vi "禹山溶解氧校准.vi"() -> ()   [LabVIEW 2016, in "斯坦道多参数.lvlib"]
uses:
  <vilib>/Utility/miscctls.llb/LVPointTypeDef.ctl
  <vilib>/Analysis/NI_AALBase.lvlib
  <vilib>/Analysis/NI_AALPro.lvlib
  <vilib>/Utility/config.llb/NI_LVConfig.lvlib
panel:
  in  "盐度自动获取":bool
  in  "大气压补偿":dbl
  in  "盐度补偿":dbl
  out "DO %":dbl caption="饱和度值"
  out "第二点校准值":dbl
  out "第一点校准值":dbl
  out "最小值":sgl format="%.2g"
  out "最大值":sgl format="%.2g"
  in  "校准停止":bool
  in  "校准模式":enum16{"两点校准", "单点校准"}(ring)
  in  "标液2":dbl
  in  "标液1":dbl
  out "波形图表":sgl(graph) caption="历史曲线"
  out "温度测量值":dbl caption="温度"
  out "变异系数":dbl format="%.6g"
  out "standard deviation":dbl caption="标准差" format="%0.2f"
  out "mean":dbl caption="均值" format="%0.2f"
  out "提示":string
  in  "校准启动":bool
  out "DO mg/L":dbl caption="测试值"
  out "电极斜率":dbl
  out "电极零点":dbl
  # "溶解氧电极设定"
  # "℃"
  # "%"
  # "mg/L"
  # "kPa"
  # "请选择校准模式:"
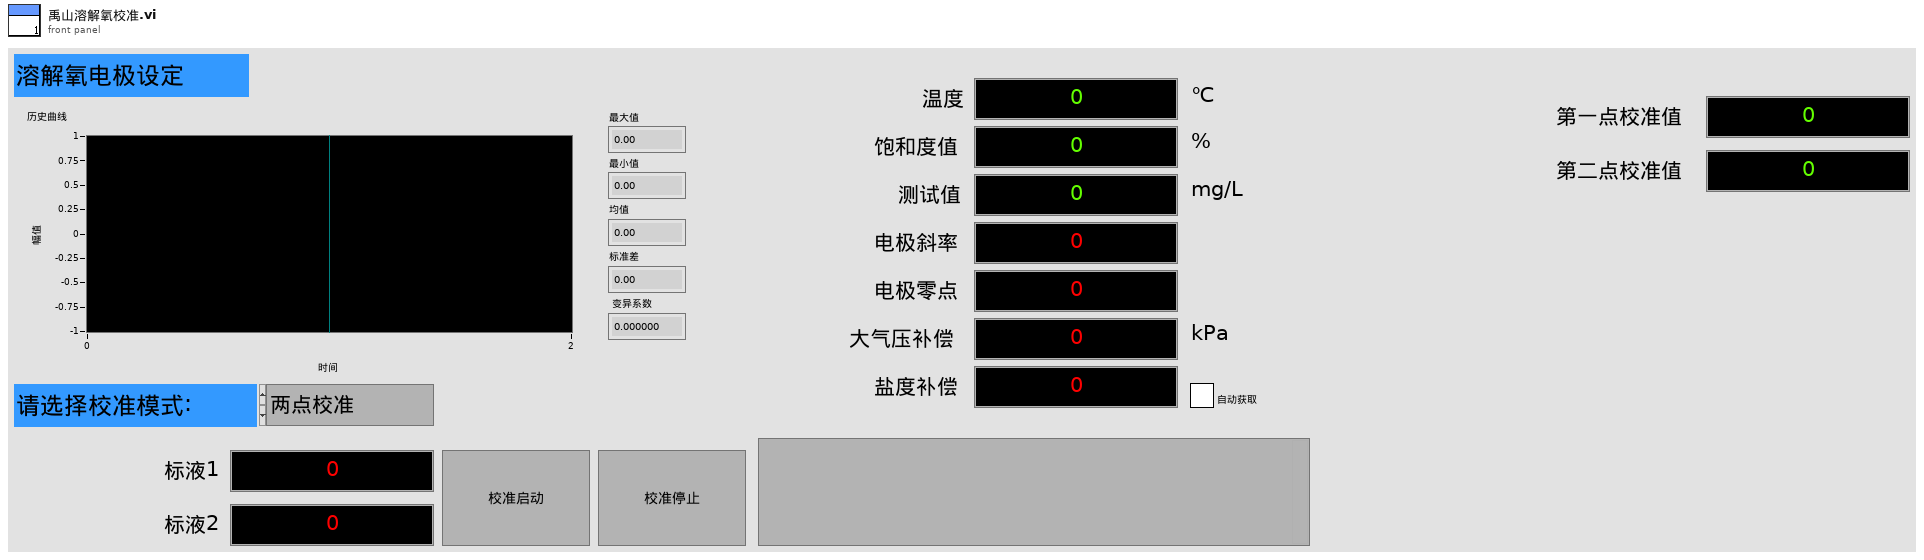
[diagram p1: front panel]
types:
  T1 = typedef "斯坦道多参数.lvlib/校准步骤.ctl" = enum16{"待机", "放置第一点标液", "第一点校准启动", "第一点校准写入", "第一点校准失败", "放置第二点标液", "第二点校准启动", "第二点校准写入", "第二点校准失败", "放置第三点标液", "第三点校准启动", "第三点校准写入", "第三点校准失败", "校准结果写入", "校准结束"}
  T2 = typedef "LVPointTypeDef.ctl" = cluster{"Horizontal":i16, "Vertical":i16}
  T3 = typedef "NI_LVConfig.lvlib/Config Data RefNum.ctl" = refnum<k1>
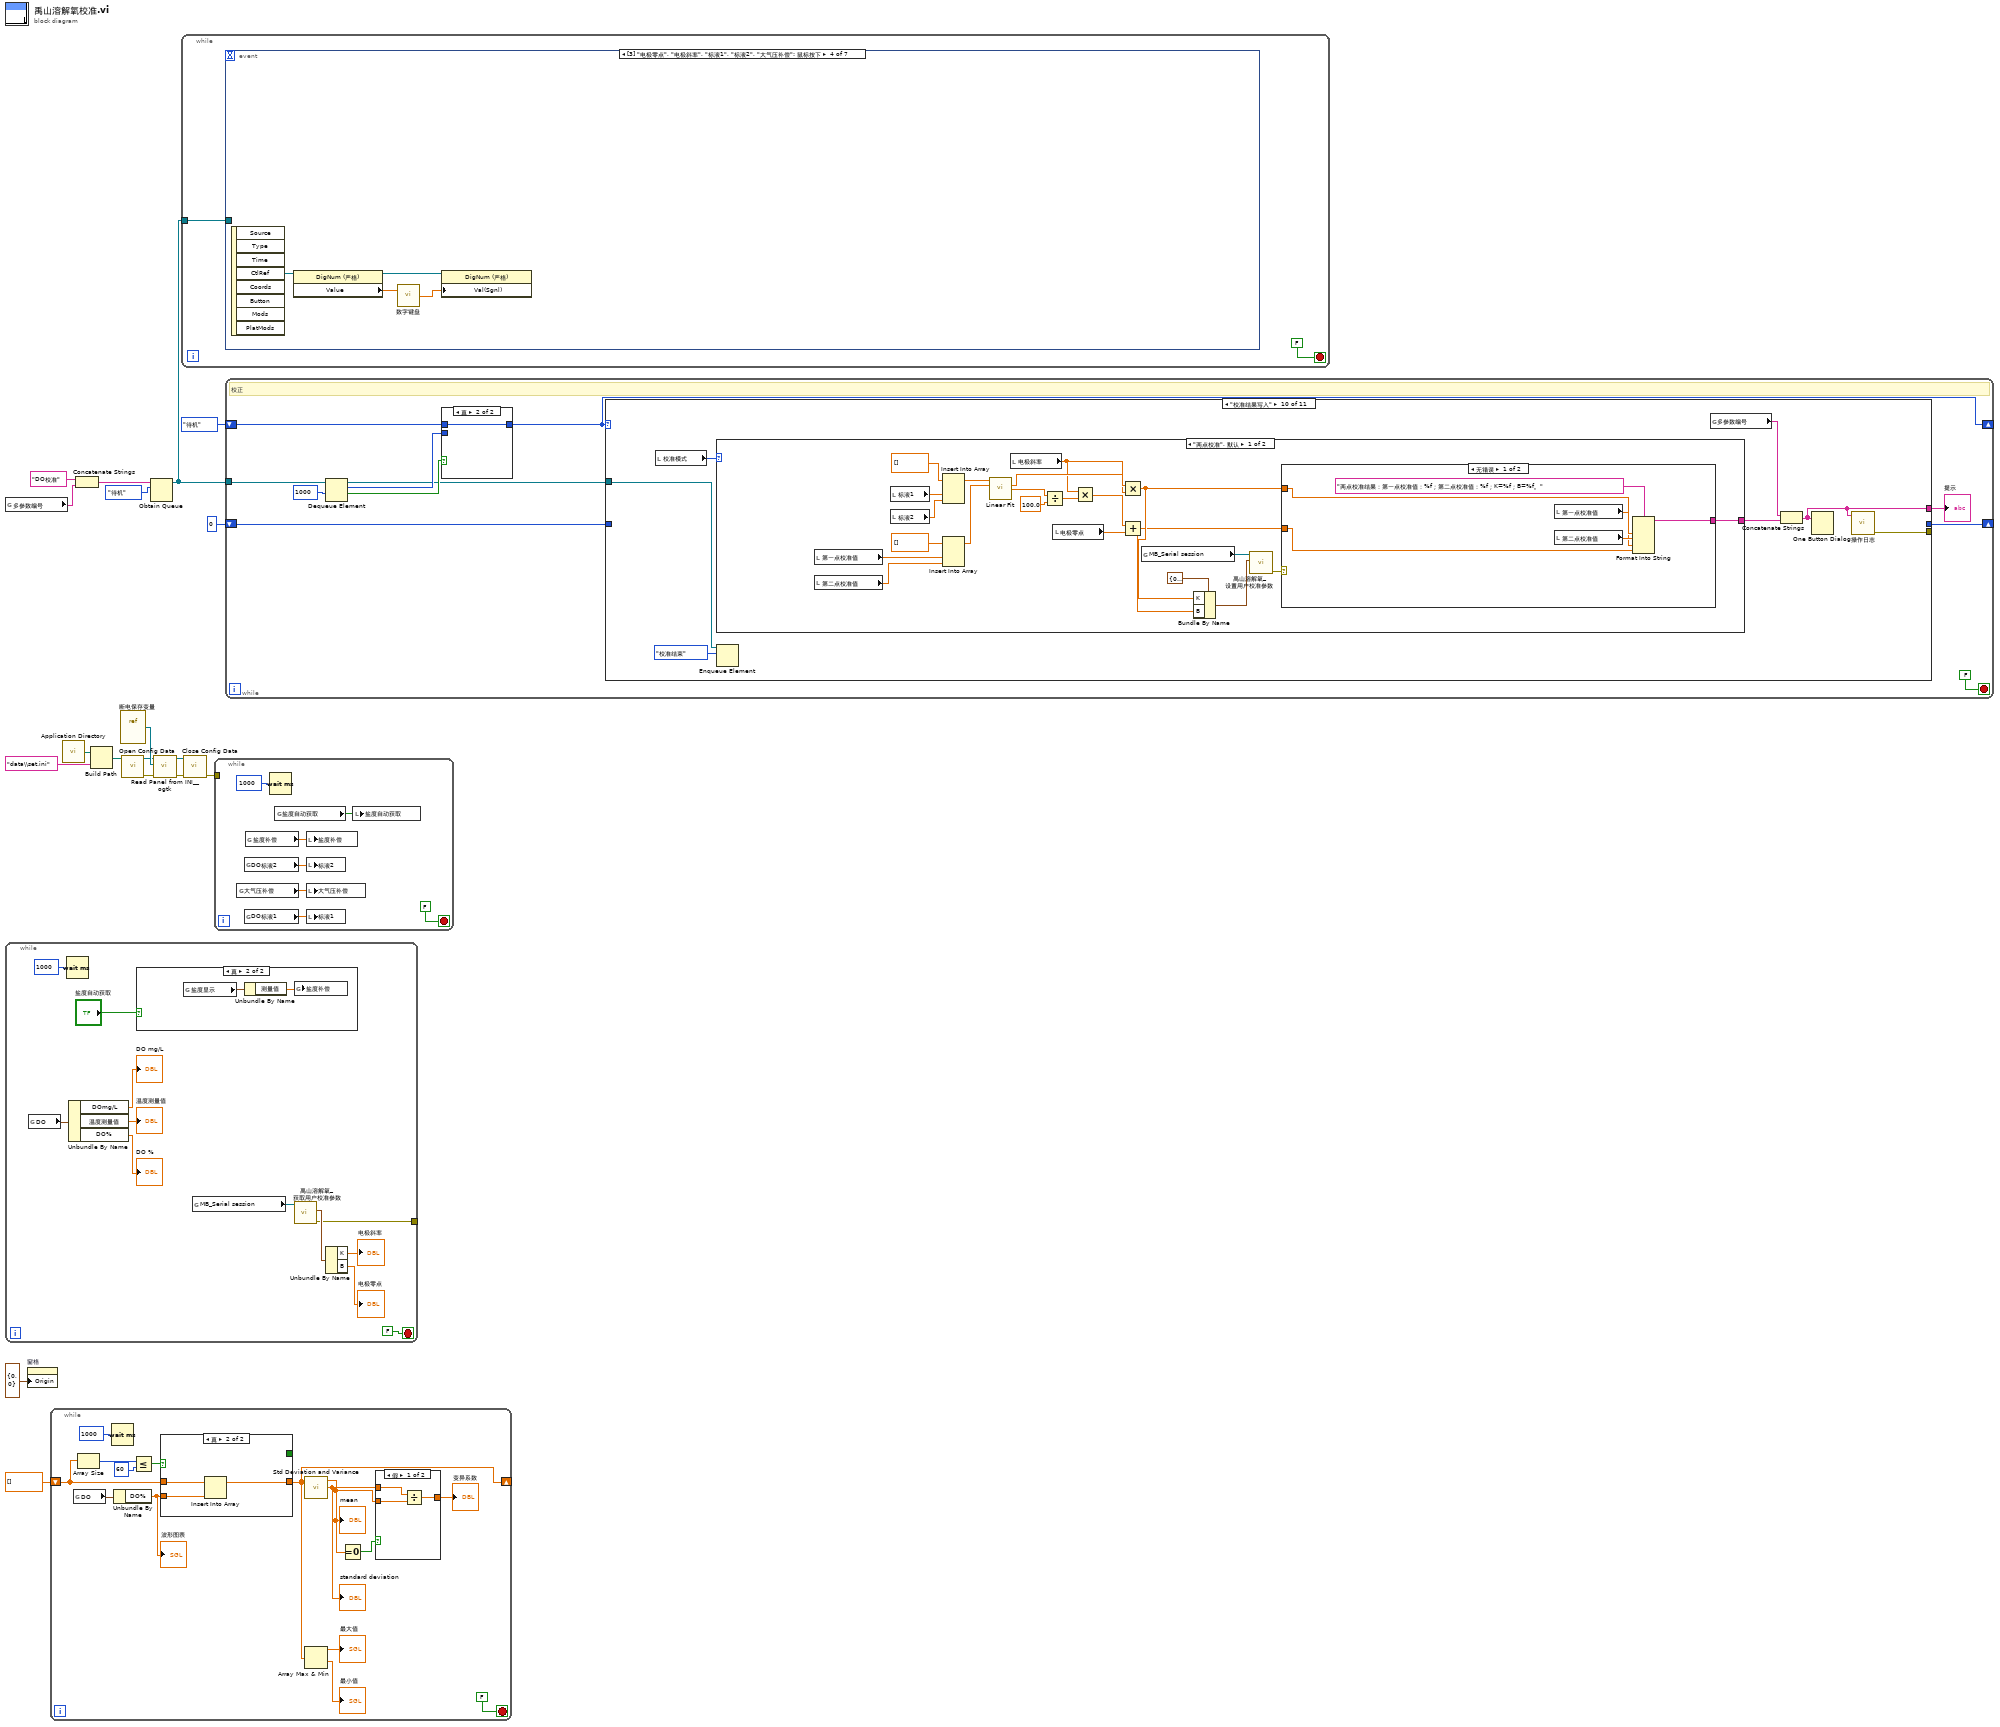
[diagram p0: block diagram]
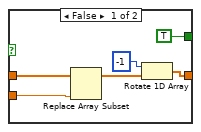
[diagram p3: hidden frame]
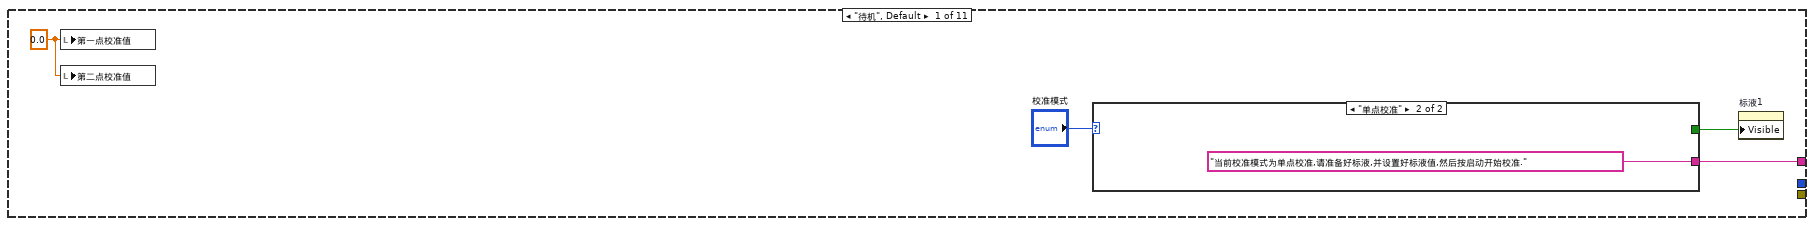
[diagram p5: hidden frame]
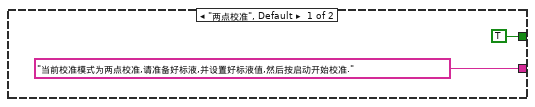
[diagram p6: hidden frame]
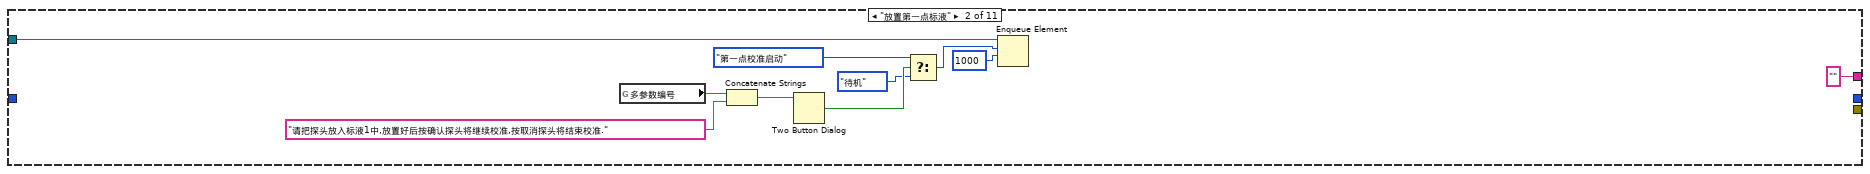
[diagram p7: hidden frame]
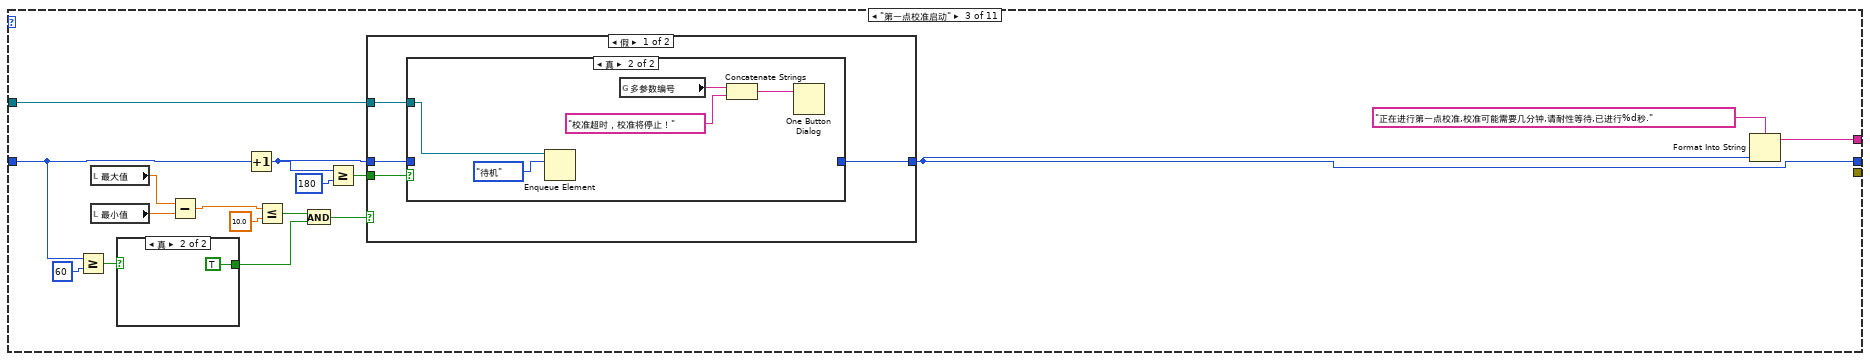
[diagram p8: hidden frame]
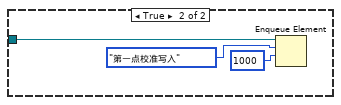
[diagram p10: hidden frame]
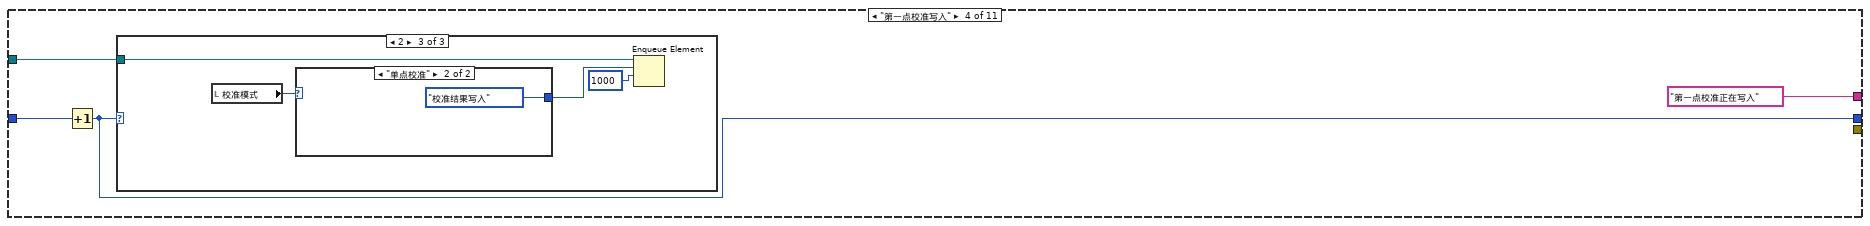
[diagram p12: hidden frame]
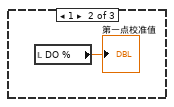
[diagram p14: hidden frame]
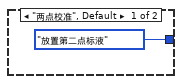
[diagram p15: hidden frame]
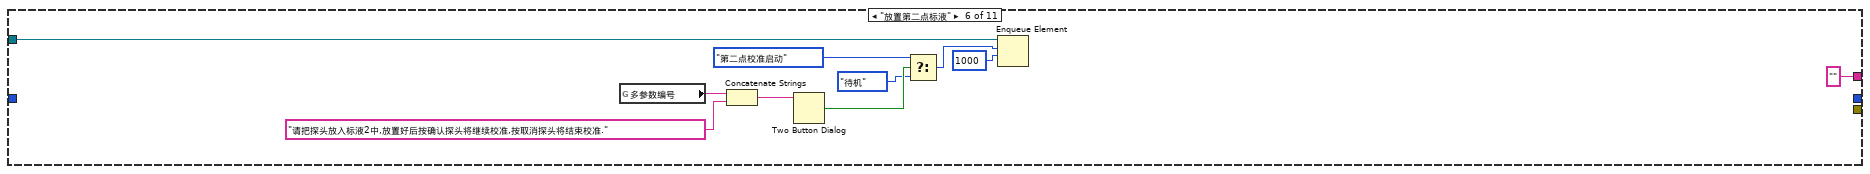
[diagram p17: hidden frame]
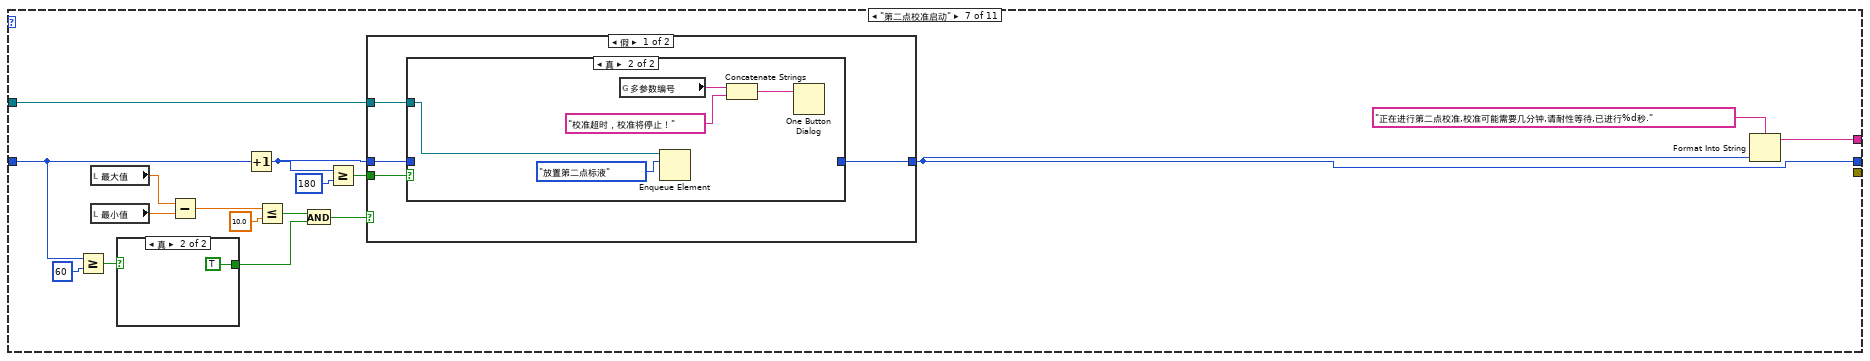
[diagram p18: hidden frame]
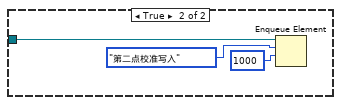
[diagram p20: hidden frame]
diagram:
  n1 = global read "多参数全局变量.vi" "多参数编号"() -> (w1:string)
  n2 = while {
    tunnel: [w25] -> _
    stop <- FALSE stop-if-true
    n3 = global read "禹山过程全局变量.vi" "DO"() -> (w22:cluster{"温度测量值":sgl, "DO%":sgl, "DOmg/L":sgl})
    n4 = Wait (ms)(milliseconds to wait=u32 1000 ("等待时间（毫秒）")) -> ()  [unwired: 1 out]
    n5 = Unbundle By Name(w22) -> ("DOmg/L"=→"DO mg/L":sgl, "温度测量值"=→"温度测量值":sgl, "DO%"=→"DO %":sgl)
    n6 = case shown="真" "盐度自动获取" {
      frame False {
      }
      frame True {
        n7 = global read "多参数全局变量.vi" "盐度显示"() -> (w32:cluster{"温度测量值":sgl, "测量值":sgl, "温度偏移修正值":sgl})
        n8 = Unbundle By Name(w32) -> ("测量值"=w31:sgl)
        n9 = global write "断电保存变量.vi" "盐度补偿"(w31) -> ()
      }
    }
    n10 = global read "多参数全局变量.vi" "MB_Serial session"() -> (w21:refnum<class "MB_Master_Serial.lvclass">)
    n11 = call "禹山溶解氧_获取用户校准参数.vi"("MB_Serial session in"=w21) -> ("error out"=w25:errorcluster, "输出值"=w28:cluster{"K":sgl, "B":sgl})  [unwired: 8 in, 1 out]
    n12 = Unbundle By Name(w28) -> ("K"=→"电极斜率":sgl, "B"=→"电极零点":sgl)
  }
  n13 = property on="窗格" class="Pane"("Origin"=T2 {"Horizontal"=0, "Vertical"=0} ("原点")) -> ()  [unwired: 2 in, 2 out]
  n14 = while {
    shift-right: [w35] -> _
    shift-left: sgl[] [] -> [w43]
    stop <- FALSE stop-if-true
    n15 = global read "禹山过程全局变量.vi" "DO"() -> (w37:cluster{"温度测量值":sgl, "DO%":sgl, "DOmg/L":sgl})
    n16 = Array Size(array=w43) -> (size(s)=w45:i32)
    n17 = Wait (ms)(milliseconds to wait=u32 1000 ("等待时间（毫秒）")) -> ()  [unwired: 1 out]
    n18 = Unbundle By Name(w37) -> ("DO%"=w36:sgl)
    "波形图表" <- w36
    n19 = Less Or Equal?(x=w45, y=60) -> (x <= y?=w44:bool)
    n20 = case shown="真" w44 {
      tunnel: w43 -> [w56 w59]
      tunnel: w36 -> [w54 w58]
      tunnel: [w52 w57] -> w35
      tunnel: [TRUE _] -> _
      frame False {
        n21 = Replace Array Subset(array=w56, new element=w54) -> (w55:sgl[])  [unwired: 1 in]
        n22 = Rotate 1D Array(1:w55, 2:-1 ("n")) -> (0:w52:sgl[])
      }
      frame True {
        n23 = Insert Into Array(array=w59, new element=w58) -> (w57:sgl[])  [unwired: 1 in]
      }
    }
    n24 = call <vilib>:"Std Deviation and Variance.vi"("X"=w35) -> ("mean"=w38:dbl, "standard deviation"=w39:dbl)  [unwired: 1 in, 1 out]
    "standard deviation" <- w39
    "mean" <- w38
    n25 = Array Max & Min(array=w35) -> (max value=→"最大值":sgl, min value=→"最小值":sgl)  [unwired: 2 out]
    n26 = Equal To 0?(x=w38) -> (x = 0?=w42:bool)
    n27 = case shown="假" w42 {
      tunnel: w39 -> [w50 _]
      tunnel: [w49 _] -> w41
      tunnel: w38 -> [w48 _]
      frame False {
        n28 = Divide(x=w50, y=w48) -> (x/y=w49:dbl)
      }
      frame True {
      }
    }
    "变异系数" <- w41
  }
  n29 = call <vilib>:"Application Directory.vi"() -> ("Application Directory"=w9:path)
  n30 = Concatenate Strings("DO校准" ("名称（未命名）"), w1) -> (w2:string)
  n31 = Build Path(base path=w9, name or relative path="data\\set.ini" ("名称或相对路径")) -> (appended path=w10:path)
  n32 = vi-ref "断电保存变量.vi"() -> (w12:refnum<vi>)
  n33 = call <vilib>:"Open Config Data.vi"("configuration file path"=w10) -> ("error out"=w6:errorcluster, "refnum"=w5:T3)  [unwired: 8 in, 1 out]
  n34 = Obtain Queue(name (unnamed)=w2, element data type=校准步骤."待机" ("枚举")) -> (queue out=w13:refnum<queue>)  [unwired: 3 in, 2 out]
  n35 = call <userlib>:"Read Panel from INI__ogtk.vi"("error in (no error)"=w6, "VI ref"=w12, "refnum"=w5) -> ("error out"=w8:errorcluster, "refnum out"=w7:T3)  [unwired: 7 in]
  n36 = while {
    tunnel: w13 -> [w60]
    stop <- FALSE stop-if-true
    n37 = event shown="[3] \"电极零点\", \"电极斜率\", \"标液1\", \"标液2\", \"大气压补偿\": 鼠标按下" {
      selector: _ -> [_ _ _ _ _ _ _]
      dyn-events: _ -> [_ _ _ _ _ _ _]
      timeout: _ -> [_ _ _ _ _ _ _]
      tunnel: w60 -> [_ w64 w70 _ _ _ _]
      event Timeout {
        n38 = event-data() -> ()  [unwired: 1 in, 3 out]
      }
      event "校准启动": Value Change {
        n39 = event-data() -> ()  [unwired: 1 in, 6 out]
        n40 = local read "校准模式"() -> (w63:enum16{"两点校准", "单点校准"})
        n41 = case shown="\"两点校准\", 默认" w63 {
          tunnel: [校准步骤."放置第一点标液" ("元素") 校准步骤."放置第二点标液" ("元素")] -> w62
          frame "两点校准", Default {
          }
          frame "单点校准" {
          }
        }
        n42 = Enqueue Element(queue=w64, element=w62) -> ()  [unwired: 2 in, 3 out]
      }
      event "校准停止": Value Change {
        n43 = event-data() -> ()  [unwired: 1 in, 6 out]
        n44 = Flush Queue(queue=w70) -> (queue out=w67:refnum<queue>)  [unwired: 1 in, 2 out]
        n45 = Enqueue Element(queue=w67, element=校准步骤."待机" ("元素"), timeout in ms (-1)=1000 ("超时毫秒(-1)")) -> ()  [unwired: 1 in, 3 out]
      }
      event "电极零点", "电极斜率", "标液1", "标液2", "大气压补偿": Mouse Down {
        n46 = event-data() -> ("CtlRef"=w71:refnum<vi>)  [unwired: 1 in, 7 out]
        n47 = property class="DigNum (严格)"(reference=w71) -> (reference out=w72:refnum<vi>, "Value"=w73:dbl)  [unwired: 1 in, 1 out]
        n48 = call "数字键盘.vi"("OldNumber"=w73) -> ("NewNumber"=w74:dbl)  [unwired: 1 in]
        n49 = property class="DigNum (严格)"(reference=w72, "Val(Sgnl)"=w74) -> ()  [unwired: 1 in, 2 out]
      }
      event "盐度补偿": Mouse Down {
        n50 = event-data() -> ("CtlRef"=w76:refnum<vi>)  [unwired: 1 in, 7 out]
        n51 = local read "盐度自动获取"() -> (w75:bool)
        n52 = case shown="假" w75 {
          tunnel: w76 -> [w77 _]
          frame False {
            n53 = property class="DigNum (严格)"(reference=w77) -> (reference out=w78:refnum<vi>, "Value"=w79:dbl)  [unwired: 1 in, 1 out]
            n54 = call "数字键盘.vi"("OldNumber"=w79) -> ("NewNumber"=w80:dbl)  [unwired: 1 in]
            n55 = property class="DigNum (严格)"(reference=w78, "Val(Sgnl)"=w80) -> ()  [unwired: 1 in, 2 out]
          }
          frame True {
          }
        }
      }
      event "电极零点", "电极斜率": Value Change {
        n56 = event-data() -> ()  [unwired: 1 in, 6 out]
        n57 = local read "电极斜率"() -> (w83:dbl)
        n58 = local read "电极零点"() -> (w82:dbl)
        n59 = global read "多参数全局变量.vi" "MB_Serial session"() -> (w81:refnum<class "MB_Master_Serial.lvclass">)
        n60 = Bundle By Name(cluster=cluster{"K":sgl, "B":sgl} {"K"=0.0, "B"=0.0} ("用户校准参数"), "K"=w83, "B"=w82) -> (w84:cluster{"K":sgl, "B":sgl})
        n61 = call "禹山溶解氧_设置用户校准参数.vi"("用户校准参数"=w84, "MB_Serial session in"=w81) -> ()  [unwired: 8 in, 2 out]
      }
      event "标液1", "标液2", "盐度补偿", "大气压补偿", "盐度自动获取": Value Change {
        n62 = event-data() -> ()  [unwired: 1 in, 6 out]
        n63 = flat-sequence {
          frame #0 {
            n64 = local read "盐度自动获取"() -> (w86:bool)
            n65 = global write "断电保存变量.vi" "DO标液2"("标液2") -> ()
            n66 = global write "断电保存变量.vi" "盐度补偿"("盐度补偿") -> ()
            n67 = global write "断电保存变量.vi" "DO标液1"("标液1") -> ()
            n68 = global write "断电保存变量.vi" "大气压补偿"("大气压补偿") -> ()
            n69 = global write "断电保存变量.vi" "盐度自动获取"(w86) -> ()
          }
          frame #1 {
            n70 = call <vilib>:"Application Directory.vi"() -> ("Application Directory"=w100:path)
            n71 = Build Path(base path=w100, name or relative path="data\\set.ini" ("名称或相对路径")) -> (appended path=w99:path)
            n72 = call <vilib>:"Open Config Data.vi"("configuration file path"=w99) -> ("error out"=w103:errorcluster, "refnum"=w104:T3)  [unwired: 8 in, 1 out]
            n73 = vi-ref "断电保存变量.vi"() -> (w97:refnum<vi>)
            n74 = call <userlib>:"Write Panel to INI__ogtk.vi"("error in (no error)"=w103, "VI ref"=w97, "refnum"=w104) -> ("error out"=w101:errorcluster, "refnum out"=w102:T3)  [unwired: 7 in]
            n75 = call <vilib>:"Close Config Data.vi"("error in (no error)"=w101, "refnum"=w102) -> ("error out"=w93:errorcluster, "file path"=w94:path)  [unwired: 8 in]
            n76 = Open/Create/Replace File(file path (use dialog)=w94, error in=w93) -> (refnum out=w95:refnum<file>, error out=w96:errorcluster)  [unwired: 4 in, 1 out]
            n77 = Flush File(refnum=w95, error in=w96) -> (refnum out=w91:refnum<file>, error out=w92:errorcluster)
            n78 = Close File(refnum=w91, error in=w92) -> ()  [unwired: 2 out]
          }
        }
      }
    }
  }
  n79 = call <vilib>:"Close Config Data.vi"("error in (no error)"=w8, "refnum"=w7) -> ("error out"=w4:errorcluster)  [unwired: 8 in, 1 out]
  n80 = while {
    tunnel: w4 -> [_]
    stop <- FALSE stop-if-true
    n81 = global read "断电保存变量.vi" "大气压补偿"() -> (w107:dbl)
    n82 = global read "断电保存变量.vi" "DO标液2"() -> (w108:dbl)
    n83 = global read "断电保存变量.vi" "DO标液1"() -> (w109:dbl)
    n84 = global read "断电保存变量.vi" "盐度补偿"() -> (w105:dbl)
    n85 = Wait (ms)(milliseconds to wait=u32 1000 ("等待时间（毫秒）")) -> ()  [unwired: 1 out]
    n86 = global read "断电保存变量.vi" "盐度自动获取"() -> (w106:bool)
    n87 = local write "盐度补偿"(w105) -> ()
    n88 = local write "标液2"(w108) -> ()
    n89 = local write "大气压补偿"(w107) -> ()
    n90 = local write "标液1"(w109) -> ()
    n91 = local write "盐度自动获取"(w106) -> ()
  }
  n92 = while "While循环" {
    shift-right: [w113] -> _
    shift-left: 校准步骤."待机" ("枚举") -> [w114]
    shift-right: [w120] -> _
    shift-left: 0 -> [w121]
    tunnel: w13 -> [w118]
    stop <- FALSE stop-if-true
    # "校正"
    n93 = Dequeue Element(queue=w118, timeout in ms (-1)=1000 ("超时毫秒(-1)")) -> (queue out=w112:refnum<queue>, element=w115:T1, timed out?=w116:bool)  [unwired: 1 in, 1 out]
    n94 = case shown="真" w116 {
      tunnel: w115 -> [w123 _]
      tunnel: [w123 w124] -> w113
      tunnel: w114 -> [_ w124]
      frame False {
      }
      frame True {
      }
    }
    n95 = case shown="\"校准结果写入\"" w113 {
      tunnel: [w128 "" ("提示") w157 "第一点校准正在写入" ("提示") _ "" ("提示") w209 "第二点校准正在写入" ("提示") _ w234 w286] -> w119
      tunnel: w121 -> [_ _ w151 w175 _ _ w203 w227 _ _ _]
      tunnel: [_ _ w142 w174 _ _ w194 w226 _ _ _] -> w120
      tunnel: w112 -> [_ w140 w145 w173 _ w192 w197 w225 _ w238 _]
      tunnel: [_ _ _ _ _ _ _ _ _ w233 _] -> _
      frame "待机", Default {
        w125 = 0.0 ("第一点校准值")
        n96 = local write "第一点校准值"(w125) -> ()
        n97 = local write "第二点校准值"(w125) -> ()
        n98 = case shown="\"单点校准\"" "校准模式" {
          tunnel: ["当前校准模式为两点校准,请准备好标液,并设置好标液值,然后按启动开始校准." ("提示") "当前校准模式为单点校准,请准备好标液,并设置好标液值,然后按启动开始校准." ("提示")] -> w128
          tunnel: [TRUE ("可见") _] -> w126
          frame "两点校准", Default {
          }
          frame "单点校准" {
          }
        }
        n99 = property on="标液1" class="DigNum (严格)"("Visible"=w126) -> ()  [unwired: 2 in, 2 out]
      }
      frame "放置第一点标液" {
        n100 = global read "多参数全局变量.vi" "多参数编号"() -> (w132:string)
        n101 = Concatenate Strings(w132, "请把探头放入标液1中,放置好后按确认探头将继续校准,按取消探头将结束校准." ("消息")) -> (w133:string)
        n102 = Two Button Dialog(message=w133) -> (T button?=w138:bool)  [unwired: 2 in]
        n103 = Select(t=校准步骤."第一点校准启动" ("元素"), s=w138, f=校准步骤."待机" ("元素")) -> (s? t:f=w135:T1)
        n104 = Enqueue Element(queue=w140, element=w135, timeout in ms (-1)=1000 ("超时毫秒(-1)")) -> ()  [unwired: 1 in, 3 out]
      }
      frame "第一点校准启动" {
        n105 = Greater Or Equal?(x=w151, y=60) -> (x >= y?=w152:bool)
        n106 = local read "最大值"() -> (w148:sgl)
        n107 = local read "最小值"() -> (w149:sgl)
        n108 = case shown="真" w152 {
          tunnel: [_ TRUE] -> w150
          frame False {
          }
          frame True {
          }
        }
        n109 = Subtract(x=w148, y=w149) -> (x-y=w147:sgl)
        n110 = Increment(x=w151) -> (x+1=w143:i32)
        n111 = Less Or Equal?(x=w147, y=10.0) -> (x <= y?=w155:bool)
        n112 = And(x=w155, y=w150) -> (x .and. y?=w146:bool)
        n113 = Greater Or Equal?(x=w143, y=180) -> (x >= y?=w144:bool)
        n114 = case shown="假" w146 {
          tunnel: w145 -> [w161 w171]
          tunnel: w144 -> [w162 _]
          tunnel: w143 -> [w160 _]
          tunnel: [w159 _] -> w142
          frame False {
            n115 = case shown="真" w162 {
              tunnel: w161 -> [_ w168]
              tunnel: w160 -> [w163 _]
              tunnel: [w163 _] -> w159
              frame False {
              }
              frame True {
                n116 = Enqueue Element(queue=w168, element=校准步骤."待机" ("元素")) -> ()  [unwired: 2 in, 3 out]
                n117 = global read "多参数全局变量.vi" "多参数编号"() -> (w164:string)
                n118 = Concatenate Strings(w164, "校准超时，校准将停止！" ("消息")) -> (w165:string)
                n119 = One Button Dialog(message=w165) -> ()  [unwired: 1 in, 1 out]
              }
            }
          }
          frame True {
            n120 = Enqueue Element(queue=w171, element=校准步骤."第一点校准写入" ("元素"), timeout in ms (-1)=1000 ("超时毫秒(-1)")) -> ()  [unwired: 1 in, 3 out]
          }
        }
        n121 = Format Into String(format string="正在进行第一点校准,校准可能需要几分钟,请耐性等待,已进行%d秒." ("格式字符串"), w142) -> (resulting string=w157:string)  [unwired: 2 in, 1 out]
      }
      frame "第一点校准写入" {
        n122 = Increment(x=w175) -> (x+1=w174:i32)
        n123 = case shown="2" w174 {
          tunnel: w173 -> [_ _ w181]
          frame 0, Default {
          }
          frame 1 {
            n124 = local read "DO %"() -> (→"第一点校准值":dbl)
          }
          frame 2 {
            n125 = local read "校准模式"() -> (w180:enum16{"两点校准", "单点校准"})
            n126 = case shown="\"单点校准\"" w180 {
              tunnel: [校准步骤."放置第二点标液" ("元素") 校准步骤."校准结果写入" ("元素")] -> w179
              frame "两点校准", Default {
              }
              frame "单点校准" {
              }
            }
            n127 = Enqueue Element(queue=w181, element=w179, timeout in ms (-1)=1000 ("超时毫秒(-1)")) -> ()  [unwired: 1 in, 3 out]
          }
        }
      }
      frame "第一点校准失败" {
      }
      frame "放置第二点标液" {
        n128 = global read "多参数全局变量.vi" "多参数编号"() -> (w184:string)
        n129 = Concatenate Strings(w184, "请把探头放入标液2中,放置好后按确认探头将继续校准,按取消探头将结束校准." ("消息")) -> (w185:string)
        n130 = Two Button Dialog(message=w185) -> (T button?=w190:bool)  [unwired: 2 in]
        n131 = Select(t=校准步骤."第二点校准启动" ("元素"), s=w190, f=校准步骤."待机" ("元素")) -> (s? t:f=w187:T1)
        n132 = Enqueue Element(queue=w192, element=w187, timeout in ms (-1)=1000 ("超时毫秒(-1)")) -> ()  [unwired: 1 in, 3 out]
      }
      frame "第二点校准启动" {
        n133 = Greater Or Equal?(x=w203, y=60) -> (x >= y?=w204:bool)
        n134 = local read "最大值"() -> (w200:sgl)
        n135 = local read "最小值"() -> (w201:sgl)
        n136 = case shown="真" w204 {
          tunnel: [_ TRUE] -> w202
          frame False {
          }
          frame True {
          }
        }
        n137 = Subtract(x=w200, y=w201) -> (x-y=w199:sgl)
        n138 = Increment(x=w203) -> (x+1=w195:i32)
        n139 = Less Or Equal?(x=w199, y=10.0) -> (x <= y?=w207:bool)
        n140 = And(x=w207, y=w202) -> (x .and. y?=w198:bool)
        n141 = Greater Or Equal?(x=w195, y=180) -> (x >= y?=w196:bool)
        n142 = case shown="假" w198 {
          tunnel: w197 -> [w213 w223]
          tunnel: w196 -> [w214 _]
          tunnel: w195 -> [w212 _]
          tunnel: [w211 _] -> w194
          frame False {
            n143 = case shown="真" w214 {
              tunnel: w213 -> [_ w220]
              tunnel: w212 -> [w215 _]
              tunnel: [w215 _] -> w211
              frame False {
              }
              frame True {
                n144 = global read "多参数全局变量.vi" "多参数编号"() -> (w216:string)
                n145 = Enqueue Element(queue=w220, element=校准步骤."放置第二点标液" ("元素")) -> ()  [unwired: 2 in, 3 out]
                n146 = Concatenate Strings(w216, "校准超时，校准将停止！" ("消息")) -> (w217:string)
                n147 = One Button Dialog(message=w217) -> ()  [unwired: 1 in, 1 out]
              }
            }
          }
          frame True {
            n148 = Enqueue Element(queue=w223, element=校准步骤."第二点校准写入" ("元素"), timeout in ms (-1)=1000 ("超时毫秒(-1)")) -> ()  [unwired: 1 in, 3 out]
          }
        }
        n149 = Format Into String(format string="正在进行第二点校准,校准可能需要几分钟,请耐性等待,已进行%d秒." ("格式字符串"), w194) -> (resulting string=w209:string)  [unwired: 2 in, 1 out]
      }
      frame "第二点校准写入" {
        n150 = Increment(x=w227) -> (x+1=w226:i32)
        n151 = case shown="2" w226 {
          tunnel: w225 -> [_ _ w232]
          frame 0, Default {
          }
          frame 1 {
            n152 = local read "DO %"() -> (→"第二点校准值":dbl)
          }
          frame 2 {
            n153 = Enqueue Element(queue=w232, element=校准步骤."校准结果写入" ("元素"), timeout in ms (-1)=1000 ("超时毫秒(-1)")) -> ()  [unwired: 1 in, 3 out]
          }
        }
      }
      frame "第二点校准失败" {
      }
      frame "校准结果写入" {
        n154 = local read "校准模式"() -> (w236:enum16{"两点校准", "单点校准"})
        n155 = case shown="\"两点校准\", 默认" w236 {
          tunnel: [w249 w275] -> w239
          frame "两点校准", Default {
            n156 = local read "第一点校准值"() -> (w260:dbl)
            n157 = local read "第二点校准值"() -> (w259:dbl)
            n158 = local read "标液1"() -> (w257:dbl)
            n159 = local read "标液2"() -> (w256:dbl)
            n160 = Insert Into Array(array=dbl[] [] ("Weight"), new element #1=w257, new element #2=w256) -> (w255:dbl[])  [unwired: 1 in]
            n161 = Insert Into Array(array=dbl[] [] ("Weight"), new element #1=w260, new element #2=w259) -> (w254:dbl[])  [unwired: 1 in]
            n162 = call <vilib>:"Linear Fit.vi"("Y"=w255, "X"=w254) -> ("slope"=w248:dbl, "intercept"=w245:dbl)  [unwired: 9 in, 3 out]
            n163 = local read "电极斜率"() -> (w246:dbl)
            n164 = Divide(x=w245, y=100.0) -> (x/y=w241:dbl)
            n165 = local read "电极零点"() -> (w243:dbl)
            n166 = Multiply(x=w246, y=w241) -> (x*y=w244:dbl)
            n167 = Multiply(x=w248, y=w246) -> (x*y=w247:dbl)
            n168 = Add(x=w244, y=w243) -> (x+y=w242:dbl)
            n169 = global read "多参数全局变量.vi" "MB_Serial session"() -> (w253:refnum<class "MB_Master_Serial.lvclass">)
            n170 = Bundle By Name(cluster=cluster{"K":sgl, "B":sgl} {"K"=0.0, "B"=0.0} ("用户校准参数"), "K"=w247, "B"=w242) -> (w252:cluster{"K":sgl, "B":sgl})
            n171 = call "禹山溶解氧_设置用户校准参数.vi"("用户校准参数"=w252, "MB_Serial session in"=w253) -> ("error out"=w250:errorcluster)  [unwired: 8 in, 1 out]
            n172 = case shown="无错误" w250 {
              tunnel: w247 -> [w264 _]
              tunnel: w242 -> [w263 _]
              tunnel: [w262 "校准失败"] -> w249
              frame No Error {
                n173 = local read "第一点校准值"() -> (w266:dbl)
                n174 = local read "第二点校准值"() -> (w267:dbl)
                n175 = Format Into String(format string="两点校准结果：第一点校准值：%f；第二点校准值：%f；K=%f；B=%f。" ("提示"), w266, w267, w264, w263) -> (resulting string=w262:string)  [unwired: 2 in, 1 out]
              }
              frame Error {
              }
            }
          }
          frame "单点校准" {
            n176 = local read "第二点校准值"() -> (w273:dbl)
            n177 = local read "标液2"() -> (w272:dbl)
            n178 = local read "电极斜率"() -> (w270:dbl)
            n179 = Divide(x=w273, y=w272) -> (x/y=w269:dbl)
            n180 = local read "电极零点"() -> (w274:dbl)
            n181 = Divide(x=w270, y=w269) -> (x/y=w271:dbl)
            n182 = global read "多参数全局变量.vi" "MB_Serial session"() -> (w279:refnum<class "MB_Master_Serial.lvclass">)
            n183 = Bundle By Name(cluster=cluster{"K":sgl, "B":sgl} {"K"=0.0, "B"=0.0} ("用户校准参数"), "K"=w271, "B"=w274) -> (w278:cluster{"K":sgl, "B":sgl})
            n184 = call "禹山溶解氧_设置用户校准参数.vi"("用户校准参数"=w278, "MB_Serial session in"=w279) -> ("error out"=w276:errorcluster)  [unwired: 8 in, 1 out]
            n185 = case shown="无错误" w276 {
              tunnel: w271 -> [w282 _]
              tunnel: w274 -> [w281 _]
              tunnel: [w280 "校准失败"] -> w275
              frame No Error {
                n186 = local read "第二点校准值"() -> (w284:dbl)
                n187 = Format Into String(format string="单点校准结果：第二点校准值：%f；K=%f；B=%f。" ("提示"), w284, w282, w281) -> (resulting string=w280:string)  [unwired: 2 in, 1 out]
              }
              frame Error {
              }
            }
          }
        }
        n188 = Enqueue Element(queue=w238, element=校准步骤."校准结束" ("元素")) -> ()  [unwired: 2 in, 3 out]
        n189 = global read "多参数全局变量.vi" "多参数编号"() -> (w235:string)
        n190 = Concatenate Strings(w235, w239) -> (w234:string)
        n191 = One Button Dialog(message=w234) -> ()  [unwired: 1 in, 1 out]
        n192 = call "操作日志.vi"("日志信息"=w234) -> ("error out"=w233:errorcluster)  [unwired: 10 in]
      }
      frame "校准结束" {
        n193 = local read "提示"() -> (w286:string)
      }
    }
    "提示" <- w119
  }
